vi "Validate Payload.vi"(8 "error in (no error)":errorcluster, 11 "CONNECT in":refnum<class "CONNECT.lvclass">) -> (0 "error out":errorcluster, 1 "valid?":bool, 3 "CONNECT out":refnum<class "CONNECT.lvclass">)   [LabVIEW 2013, in "CONNECT.lvclass"]
uses:
  CONNECT.lvclass
  ControlPacket/ControlPacket.lvclass
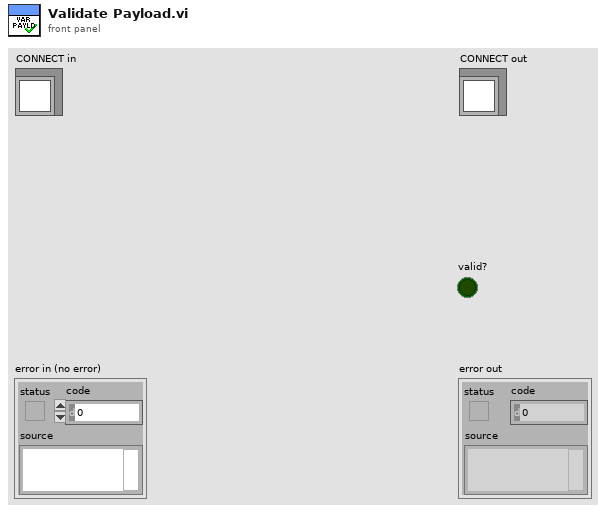
[diagram p1: front panel]
types:
  T1 = typedef "CONNECT.lvclass/ConnectFlags -- cluster.ctl" = cluster{"Reserved":bool, "Clean Session":bool, "Will Flag":bool, "Will QoS 1":bool, "Will QoS 2":bool, "Will Retain":bool, "Password Flag":bool, "User Name Flag":bool}
  T2 = typedef "CONNECT.lvclass/ConnectPayload -- cluster.ctl" = cluster{"Will Topic":string, "Will Message":string, "Username":string, "Password":string}
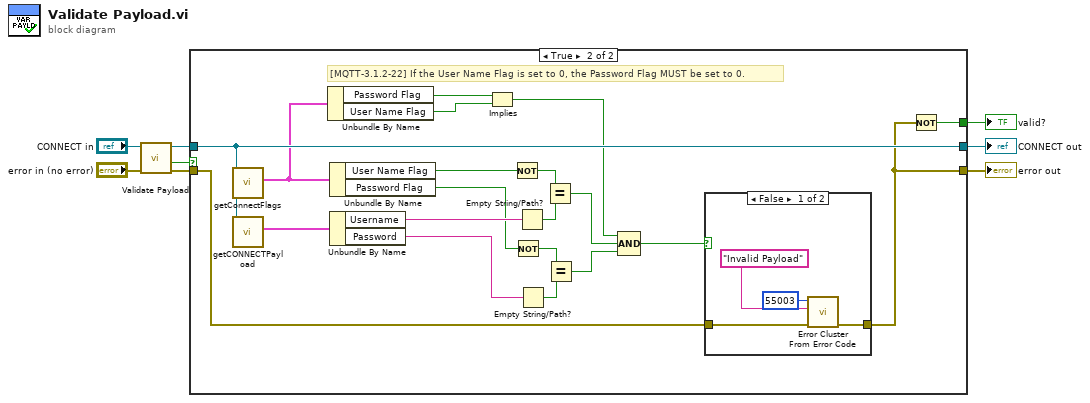
[diagram p0: block diagram]
diagram:
  n1 = call-parent "Validate Payload.vi"("error in (no error)"="error in (no error)", "ControlPacket in"="CONNECT in") -> ("error out"=w4:errorcluster, "valid?"=w6:bool, "ControlPacket out"=w5:refnum<class "CONNECT.lvclass">)  [unwired: 7 in]
  n2 = case shown="True" w6 {
    selector: w6 -> [w11 _]
    tunnel: w5 -> [w10 w31]
    tunnel: w4 -> [w9 w22]
    tunnel: [w9 w21] -> w3
    tunnel: [w10 w31] -> w2
    tunnel: [w11 w29] -> w1
    frame False {
      # "If parent calls it invalid, do not process more specific validation"
    }
    frame True {
      # "[MQTT-3.1.2-22] If the User Name Flag is set to 0, the Password Flag MUST be set to 0."
      n3 = call "getConnectFlags.vi"("CONNECT in"=w31) -> ("Connect Flags"=w15:T1)  [unwired: 9 in, 1 out]
      n4 = call "getCONNECTPayload.vi"("CONNECT in"=w31) -> ("Payload"=w30:T2)  [unwired: 9 in, 1 out]
      n5 = Unbundle By Name(w15) -> ("Password Flag"=w14:bool, "User Name Flag"=w13:bool)
      n6 = Unbundle By Name(w15) -> ("User Name Flag"=w27:bool, "Password Flag"=w18:bool)
      n7 = Unbundle By Name(w30) -> ("Username"=w28:string, "Password"=w17:string)
      n8 = Implies(1:w13, 2:w14) -> (0:w12:bool)
      n9 = Not(x=w27) -> (.not. x?=w25:bool)
      n10 = Not(x=w18) -> (.not. x?=w20:bool)
      n11 = Empty String/Path?(string/path=w28) -> (empty?=w26:bool)
      n12 = Empty String/Path?(string/path=w17) -> (empty?=w19:bool)
      n13 = Equal?(x=w25, y=w26) -> (x = y?=w24:bool)
      n14 = Equal?(x=w20, y=w19) -> (x = y?=w16:bool)
      n15 = Compound Arithmetic op=AND(w12, w24, w16) -> (w23:bool)
      n16 = case shown="False" w23 {
        tunnel: [w35 w36] -> w21
        tunnel: w22 -> [w32 w36]
        frame False {
          n17 = call <vilib>:"Error Cluster From Error Code.vi"("error in (no error)"=w32, "error message (\"\")"="Invalid Payload" ("error message (\"\")"), "error code (0)"=55003) -> ("error out"=w35:errorcluster)  [unwired: 6 in]
        }
        frame True {
        }
      }
      n18 = Not(x=w21) -> (.not. x?=w29:bool)
    }
  }
  "error out" <- w3
  "CONNECT out" <- w2
  "valid?" <- w1
